vi "Measure Output Current.vi"(8 "error":errorcluster, 11 "VISA in":refnum<visa-resource-name>) -> (0 "error out":errorcluster, 2 "Output Current":dbl format="%.4f", 3 "VISA out":refnum<visa-resource-name>)   [LabVIEW 2023, in "TDK20-38 API.lvlib"]
uses:
  TDK20-38 API.lvlib
  <userlib>/TDK-Lambda GEN LAN Series/TDK-Lambda GEN LAN Series.lvlib
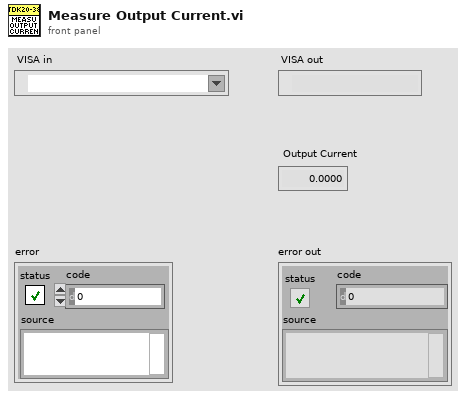
[diagram p1: front panel]
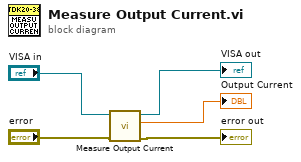
[diagram p0: block diagram]
diagram:
  n1 = call <userlib>:"Measure Output Current.vi"("error"="error", "VISA"="VISA in") -> ("error out"=→"error out":errorcluster, "Output Current"=→"Output Current":dbl, "VISA out"=→"VISA out":refnum<visa-resource-name>)  [unwired: 7 in]
